vi "Mover.vi"() -> ()   [LabVIEW 2011]
uses:
  <instrlib>/niHWS/nihws.llb/niHWS Open File Permissions ID.ctl
  <vilib>/Instr/_visa.llb/Select Event Type.ctl
  <vilib>/DAQmx/write.llb/DAQmx Write (Counter Time 1Chan 1Samp).vi
  <vilib>/DAQmx/write.llb/DAQmx Write (Digital Bool 1Line 1Point).vi
  <vilib>/DAQmx/read.llb/DAQmx Read (Analog 1D Wfm NChan NSamp).vi
  <vilib>/DAQmx/configure/timing.llb/DAQmx Timing (Sample Clock).vi
  <vilib>/DAQmx/miscellaneous.llb/DAQmx Fill In Error Info.vi
  <vilib>/addons/control/pid/pid.llb/PID Control Input Filter (DBL).vi
  <instrlib>/niHWS/nihws.llb/niHWS Write Analog WDT.vi
  <instrlib>/niHWS/nihws.llb/niHWS Write Analog DBL.vi
  <vilib>/express/express arith-compare/Formula/XNode/ExpressFormulaBlockNode.xnode
  <vilib>/ptbypt/NI_PtbyPt.lvlib
  <vilib>/addons/control/pid/NI_PID_autopid.lvlib
  <vilib>/addons/control/pid/NI_PID_pid.lvlib
panel:
  in  "x":dbl=3.0
  in  "Tab Control":enum32{"Settings", "Run"}(tab)
  in  "PID gains":T1={"proportional gain (Kc)"=0.05, "integral time (Ti, min)"=0.02, "derivative time (Td, min)"=0.0} {"derivative time (Td, min)" format="%.3f"; "integral time (Ti, min)" format="%.3f"; "proportional gain (Kc)" format="%.3f"}
  in  "Avg Samples":i32=500
  in  "VISA resource name":refnum<visa-resource-name>="Mouse"
  in  "DPI":dbl=3500.0
  in  "Frequency":dbl=30000.0
  in  "Selected Path for h5":path
  out "Speed History":dbl(graph)
  out "Speed (Inch/sec)":dbl format="%0.2f"
  in  "Target Speed":dbl format="%.2f"
  in  "stop":bool
  in  "Duty Cycle":dbl=0.1 format="%.2f"
  in  "Auto-Speed":bool
  out "SyncRead":dbl
  out "Photodiode":waveform(dbl)[](array[waveform])
  in  "SyncWrite":bool
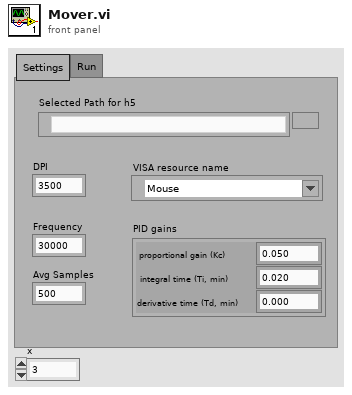
[diagram p1: front panel]
types:
  T1 = cluster{"proportional gain (Kc)":dbl, "integral time (Ti, min)":dbl, "derivative time (Td, min)":dbl}
  T2 = typedef "niHWS Open File Permissions ID.ctl" = enum32{"Read Only", "Read/Write Existing", "Read/Write/Create New", "Read/Write/Create New Always"}
  T3 = typedef "Select Event Type.ctl" = u32
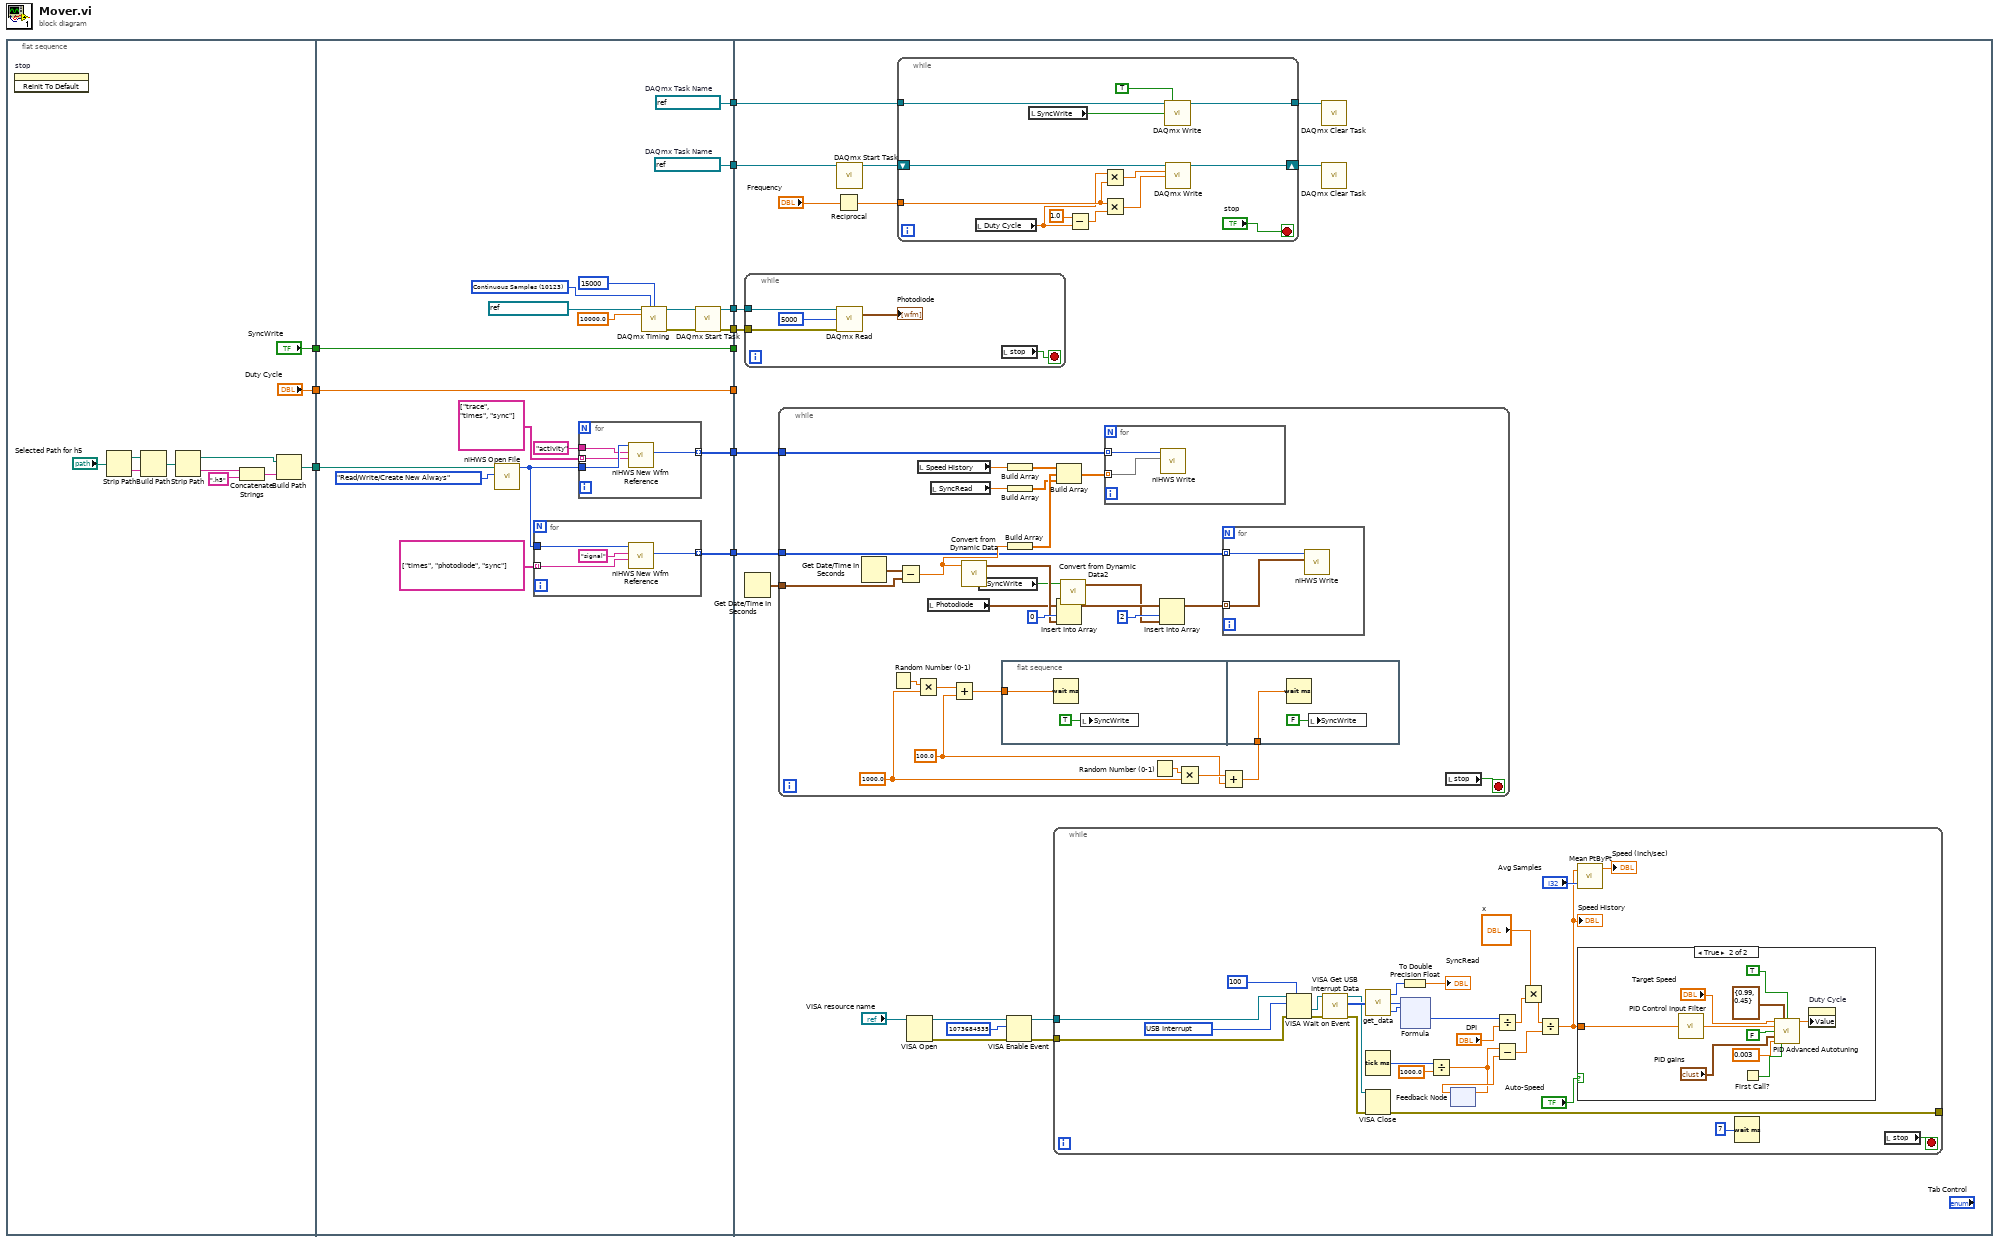
[diagram p0: block diagram]
diagram:
  n1 = flat-sequence {
    tunnel: ["SyncWrite"] -> w11
    tunnel: ["Duty Cycle"] -> w9
    tunnel: [w20] -> w3
    tunnel: w11 -> [w42]
    tunnel: [w42] -> w10
    tunnel: w9 -> [w41]
    tunnel: [w41] -> w8
    tunnel: [w36] -> w7
    tunnel: [w35] -> w6
    tunnel: [w29] -> w5
    tunnel: [w28] -> w4
    tunnel: w3 -> [w26]
    tunnel: [w24] -> w2
    tunnel: [w23] -> w1
    tunnel: w10 -> [_]
    tunnel: w8 -> [_]
    tunnel: w7 -> [w58]
    tunnel: w6 -> [w57]
    tunnel: w5 -> [w55]
    tunnel: w4 -> [w54]
    tunnel: w2 -> [w52]
    tunnel: w1 -> [w53]
    frame #0 {
      n2 = invoke on="stop" class="Bool (strict)" method="Reinit To Default"() -> ()  [unwired: 3 in, 3 out]
      n3 = Strip Path(path="Selected Path for h5") -> (stripped path=w19:path, name=w16:string)
      n4 = Build Path(base path=w19, name or relative path=w16) -> (appended path=w17:path)
      n5 = Strip Path(path=w17) -> (stripped path=w15:path, name=w13:string)
      n6 = Concatenate Strings(w13, ".h5" ("search string")) -> (w12:string)
      n7 = Build Path(base path=w15, name or relative path=w12) -> (appended path=w20:path)
    }
    frame #1 {
      w23 = refnum<k21> "DigitalSync"  # DAQmx Task Name
      w24 = refnum<k21> "PulseMotor"  # DAQmx Task Name
      w34 = 10123 items=["Finite Samples"=10178, "Continuous Samples"=10123, "Hardware Timed Single Point"=12522] ("sample mode")
      n8 = call <instrlib>:"niHWS Open File.vi"("permissions (0:read only)"=niHWS_Open_File_Permissions_ID."Read/Write/Create New Always", "file path"=w26) -> ("file handle"=w39:u32)  [unwired: 8 in, 1 out]
      n9 = for {
        tunnel: w39 -> [w49]
        tunnel: [w48] -> w35 mode=indexing
        tunnel: string[] ["times", "photodiode", "sync"] -> [w47] mode=indexing
        n10 = call <instrlib>:"niHWS New Wfm Reference.vi"("waveform name (empty)"=w47, "group name (empty)"="signal", "file handle in"=w49) -> ("waveform reference"=w48:u32)  [unwired: 6 in, 2 out]
      }
      n11 = for {
        tunnel: w39 -> [w46]
        tunnel: [w45] -> w36 mode=indexing
        tunnel: "activity" ("group name (empty)") -> [w44]
        tunnel: string[] ["trace", "times", "sync"] -> [w43] mode=indexing
        n12 = call <instrlib>:"niHWS New Wfm Reference.vi"("waveform name (empty)"=w43, "group name (empty)"=w44, "file handle in"=w46) -> ("waveform reference"=w45:u32)  [unwired: 6 in, 2 out]
      }
      n13 = call-poly <vilib>:"DAQmx Timing.vi"("task/channels in"=refnum<k21> "PhotodiodeBall", "sample mode"=w34, "samples per channel"=15000, "rate"=10000.0) -> ("task out"=w31:refnum<k21>, "error out"=w30:errorcluster)  [unwired: 10 in]
      n14 = call <vilib>:"DAQmx Start Task.vi"("task/channels in"=w31, "error in"=w30) -> ("task out"=w29:refnum<k21>, "error out"=w28:errorcluster)  [unwired: 12 in]
    }
    frame #2 {
      n15 = while {
        tunnel: w55 -> [w70]
        tunnel: w54 -> [w69]
        stop <- w73 stop-if-true
        n16 = call-poly <vilib>:"DAQmx Read.vi"("task/channels in"=w70, "number of samples per channel"=5000, "error in"=w69) -> ("data"=→"Photodiode":waveform(dbl)[])  [unwired: 10 in, 2 out]
        n17 = local read "stop"() -> (w73:bool)
      }
      n18 = Get Date/Time In Seconds() -> (seconds since 1Jan1904=w56:timestamp)
      n19 = while {
        tunnel: w58 -> [w85]
        tunnel: w57 -> [w84]
        tunnel: w56 -> [w83]
        stop <- w101 stop-if-true
        w93 = 100.0 ("y")
        w94 = 1000.0 ("y")
        n20 = Get Date/Time In Seconds() -> (seconds since 1Jan1904=w82:timestamp)
        n21 = Random Number (0-1)() -> (number: 0 to 1=w100:dbl)
        n22 = Subtract(x=w82, y=w83) -> (x-y=w92:dbl)
        n23 = Multiply(x=w100, y=w94) -> (x*y=w99:dbl)
        n24 = local read "Speed History"() -> (w86:dbl)
        n25 = local read "Photodiode"() -> (w81:waveform(dbl)[])
        n26 = local read "SyncRead"() -> (w80:dbl)
        n27 = Add(x=w99, y=w93) -> (x+y=w98:dbl)
        n28 = call "Convert from Dynamic Data"("Dynamic Data Type"=w92) -> ("Waveform"=w90:waveform(dbl))  [unwired: 3 in]
        n29 = local read "SyncWrite"() -> (w74:bool)
        n30 = flat-sequence {
          tunnel: w98 -> [w106]
          tunnel: w95 -> [w108]
          frame #0 {
            n31 = Wait (ms)(milliseconds to wait=w106) -> ()  [unwired: 1 out]
            n32 = local write "SyncWrite"(TRUE ("data")) -> ()
          }
          frame #1 {
            n33 = Wait (ms)(milliseconds to wait=w108) -> ()  [unwired: 1 out]
            n34 = local write "SyncWrite"(FALSE ("data")) -> ()
          }
        }
        n35 = Build Array(w86) -> (w89:dbl[])
        n36 = Build Array(w80) -> (w79:dbl[])
        n37 = Build Array(w92) -> (w87:dbl[])
        n38 = Build Array(w89, w87, w79) -> (w88:dbl[][])
        n39 = Insert Into Array(array=w81, index=0, new element=w90) -> (w78:waveform(dbl)[])
        n40 = call "Convert from Dynamic Data2"("Dynamic Data Type"=w74) -> ("Waveform"=w75:waveform(dbl))  [unwired: 3 in]
        n41 = for {
          tunnel: w88 -> [w105] mode=indexing
          tunnel: w85 -> [w104] mode=indexing
          n42 = call-poly <instrlib>:"niHWS Write.vi"("data"=w105, "waveform reference in"=w104) -> ()  [unwired: 8 in, 2 out]
        }
        n43 = Random Number (0-1)() -> (number: 0 to 1=w96:dbl)
        n44 = Insert Into Array(array=w78, index=2, new element=w75) -> (w76:waveform(dbl)[])
        n45 = Multiply(x=w96, y=w94) -> (x*y=w97:dbl)
        n46 = Add(x=w97, y=w93) -> (x+y=w95:dbl)
        n47 = for {
          tunnel: w84 -> [w103] mode=indexing
          tunnel: w76 -> [w102] mode=indexing
          n48 = call-poly <instrlib>:"niHWS Write.vi"("analog waveform"=w102, "waveform reference in"=w103) -> ()  [unwired: 8 in, 2 out]
        }
        n49 = local read "stop"() -> (w101:bool)
      }
      n50 = Reciprocal(x="Frequency") -> (1/x=w67:dbl)
      n51 = call <vilib>:"DAQmx Start Task.vi"("task/channels in"=w52) -> ("task out"=w51:refnum<k21>)  [unwired: 13 in, 1 out]
      n52 = while {
        tunnel: w67 -> [w170]
        shift-right: [w166] -> w66
        shift-left: w51 -> [w172]
        tunnel: w53 -> [w162]
        tunnel: [w161] -> w59
        stop <- "stop" stop-if-true
        n53 = local read "Duty Cycle"() -> (w164:dbl)
        n54 = local read "SyncWrite"() -> (w160:bool)
        n55 = Subtract(x=1.0, y=w164) -> (x-y=w169:dbl)
        n56 = Multiply(x=w164, y=w170) -> (x*y=w168:dbl)
        n57 = Multiply(x=w170, y=w169) -> (x*y=w167:dbl)
        n58 = call-poly <vilib>:"DAQmx Write.vi"("task/channels in"=w162, "auto start"=TRUE, "data"=w160) -> ("task out"=w161:refnum<k21>)  [unwired: 10 in, 2 out]
        n59 = call-poly <vilib>:"DAQmx Write.vi"("task/channels in"=w172, "high time"=w168, "low time"=w167) -> ("task out"=w166:refnum<k21>)  [unwired: 10 in, 2 out]
      }
      n60 = VISA Open(VISA resource name="VISA resource name") -> (VISA resource name=w63:refnum<visa-resource-name>, error out=w64:errorcluster)  [unwired: 1 in, 3 out]
      n61 = VISA Enable Event(8:w64, 10:u32 1073684535 ("event type"), 11:w63) -> (0:w60:errorcluster, 3:w61:refnum<visa-resource-name>)  [unwired: 1 out]
      n62 = while {
        tunnel: w61 -> [w139]
        tunnel: [w138] -> _
        tunnel: w60 -> [w130]
        stop <- w131 stop-if-true
        w122 = T3 1073684535 items=["Service Request"=1073684491, "Trigger"=3221168138, "Clear"=1073684493, "VXI Signal"=1073684512, "VXI/VME Interrupt"=3221168161, "VXI/VME Sysfail"=1073684509, "VXI/VME Sysreset"=1073684510, "GPIB CIC"=1073684498, "GPIB Talk"=1073684499, "GPIB Listen"=1073684500, "PXI Interrupt"=1073684514, "Serial Break"=1073684515, "Serial TermChar"=1073684516, "Serial CTS"=1073684521, "Serial DSR"=1073684522, "Serial DCD"=1073684524, "Serial RI"=1073684526, "Serial Character"=1073684533, "USB Interrupt"=1073684535, "All Enabled"=1073709055] ("Event Type")
        n63 = VISA Wait on Event(7:u32 100 ("timeout (0)"), 8:w130, 10:w122, 11:w139) -> (0:w134:errorcluster, 1:w133:refnum<visa-resource-name>)  [unwired: 3 out]
        n64 = call <vilib>:"VISA Get USB Interrupt Data.vi"("error in (no error)"=w134, "VISA USB Intr Event"=w133) -> ("error out"=w136:errorcluster, "data buffer"=w137:u8[], "VISA USB Intr Event out"=w135:refnum<visa-resource-name>)  [unwired: 7 out]
        n65 = call "get_data.vi"("data buffer"=w137) -> ("Click Value"=w120:i8, "X Value"=w127:i8, "Y Value"=w126:i8)
        n66 = Tick Count (ms)() -> (millisecond timer value=w116:u32)
        n67 = VISA Close(VISA resource name=w135, error in (no error)=w136) -> (error out=w138:errorcluster)
        n68 = xnode ("Formula")("X1"=w127, "X2"=w126) -> ("Result"=w118:i8)  [unwired: 1 in, 1 out]
        n69 = To Double Precision Float(number=w120) -> (double precision float=→"SyncRead":dbl)
        n70 = Divide(x=w116, y=1000.0) -> (x/y=w114:dbl)
        n71 = feedback-in #1(w114) -> ()
        n72 = feedback #1() -> (w128:dbl)  [unwired: 1 in]
        n73 = Divide(x=w118, y="DPI") -> (x/y=w112:dbl)
        n74 = Subtract(x=w114, y=w128) -> (x-y=w117:dbl)
        n75 = Multiply(x="x", y=w112) -> (x*y=w111:dbl)
        n76 = Divide(x=w111, y=w117) -> (x/y=w121:dbl)
        "Speed History" <- w121
        n77 = call <vilib>:"Mean PtByPt.vi"("x"=w121, "sample length"="Avg Samples") -> ("mean"=→"Speed (Inch/sec)":dbl)  [unwired: 2 in, 1 out]
        n78 = case shown="True" "Auto-Speed" {
          tunnel: w121 -> [_ w144]
          frame False {
          }
          frame True {
            n79 = call-poly <vilib>:"PID Control Input Filter.vi"("input"=w144) -> ("output"=w143:dbl)  [unwired: 4 in]
            n80 = First Call?() -> (First Call?: T/F=w147:bool)
            n81 = call <vilib>:"PID Advanced Autotuning.vi"("setpoint"="Target Speed", "output range"=cluster{"output high":dbl, "output low":dbl} {"output high"=0.99, "output low"=0.45}, "Auto? (F)"=TRUE, "process variable"=w143, "Autotune? (F)"=FALSE, "PID Gains"="PID gains", "dt (s)"=0.003, "reinitialize? (F)"=w147) -> ("output"=w140:dbl)  [unwired: 6 in, 1 out]
            n82 = property on="Duty Cycle" class="DigNum (strict)"("Value"=w140) -> ()  [unwired: 2 in, 2 out]
          }
        }
        n83 = Wait (ms)(milliseconds to wait=u32 7) -> ()  [unwired: 1 out]
        n84 = local read "stop"() -> (w131:bool)
      }
      n85 = call <vilib>:"DAQmx Clear Task.vi"("task in"=w59) -> ()  [unwired: 14 in, 1 out]
      n86 = call <vilib>:"DAQmx Clear Task.vi"("task in"=w66) -> ()  [unwired: 14 in, 1 out]
    }
  }
